vi "RunOperation.vi"(10 "Inputs":string[](array[string]), 11 "DiffVI in":refnum<class "DiffVI.lvclass">) -> (1 "Output/Failure":string, 2 "CLI Process Return Code":i32, 3 "DiffVI out":refnum<class "DiffVI.lvclass">)   [LabVIEW 2015, in "DiffVI.lvclass"]
uses:
  DiffVI.lvclass
  <vilib>/Utility/error.llb/DialogType.ctl
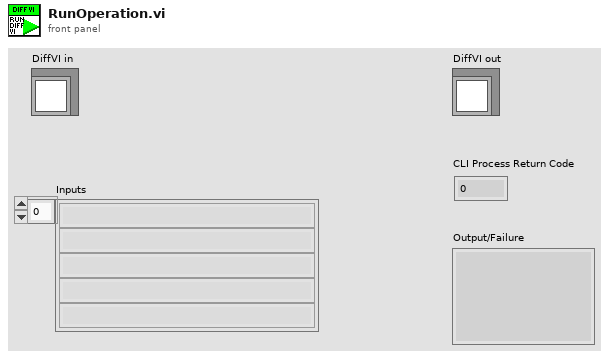
[diagram p1: front panel]
types:
  T1 = typedef "DialogType.ctl" = u16
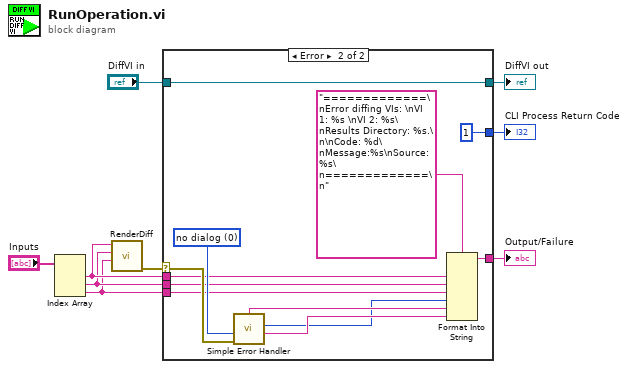
[diagram p0: block diagram]
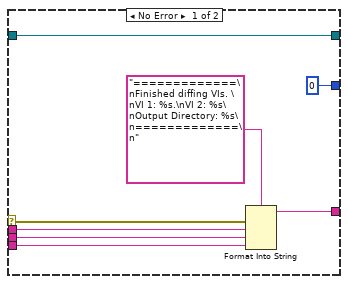
[diagram p2: hidden frame]
diagram:
  n1 = Index Array(array="Inputs") -> (element #1=w5:string, element #2=w4:string, element #3=w3:string)  [unwired: 3 in]
  n2 = call "RenderDiff.vi"("output directory"=w3, "path to old VI"=w4, "path to new VI"=w5) -> ("error out"=w6:errorcluster)  [unwired: 8 in]
  n3 = case shown="Error" w6 {
    selector: w6 -> [w16 w28]
    tunnel: [w15 w29] -> w8
    tunnel: [0 ("Exit Code (0)") 1 ("Exit Code (0)")] -> w7
    tunnel: w4 -> [w12 w20]
    tunnel: w3 -> [w11 w21]
    tunnel: w5 -> [w13 w19]
    tunnel: [w10 w18] -> w2
    tunnel: "DiffVI in" -> [w10 w18]
    frame No Error {
      n4 = Format Into String(format string="=============\nFinished diffing VIs. \nVI 1: %s.\nVI 2: %s\nOutput Directory: %s\n=============\n", error in=w16, w13, w12, w11) -> (resulting string=w15:string)  [unwired: 1 in, 1 out]
    }
    frame Error {
      w27 = T1 0 items=["no dialog", "OK message", "continue or stop message", "OK message + warnings", "continue/stop + warnings"] ("type of dialog (OK msg:1)")
      n5 = call <vilib>:"Simple Error Handler.vi"("type of dialog (OK msg:1)"=w27, "error in (no error)"=w28) -> ("code out"=w22:i32, "source out"=w23:string, "message"=w24:string)  [unwired: 3 in, 2 out]
      n6 = Format Into String(format string="=============\nError diffing VIs: \nVI 1: %s \nVI 2: %s\nResults Directory: %s.\n\nCode: %d\nMessage:%s\nSource: %s\n=============\n", w19, w20, w21, w22, w24, w23) -> (resulting string=w29:string)  [unwired: 2 in, 1 out]
    }
  }
  "DiffVI out" <- w2
  "CLI Process Return Code" <- w7
  "Output/Failure" <- w8
